vi "Estimate All Positions New.vi"(8 "Input AnchorArray":refnum<class "Anchor.lvclass">[](array[class]), 10 "Tag.lvclass":refnum<class "Tag.lvclass">) -> (2 "PositionCluster [tagID, x, y, anchorID, distances]":T2)   [LabVIEW 2014]
uses:
  Anchor/Anchor.lvclass
  Tag.lvclass
  Position.lvclass
panel:
  out "error out 3":errorcluster
  in  "error in (no error) 2":errorcluster
  out "error out 2":errorcluster
  out "TagID":dbl
  in  "error in (no error)":errorcluster
  out "Intersections":T1(array[cluster])
  # "This will be returned"
  # "Put intersection values in this control"
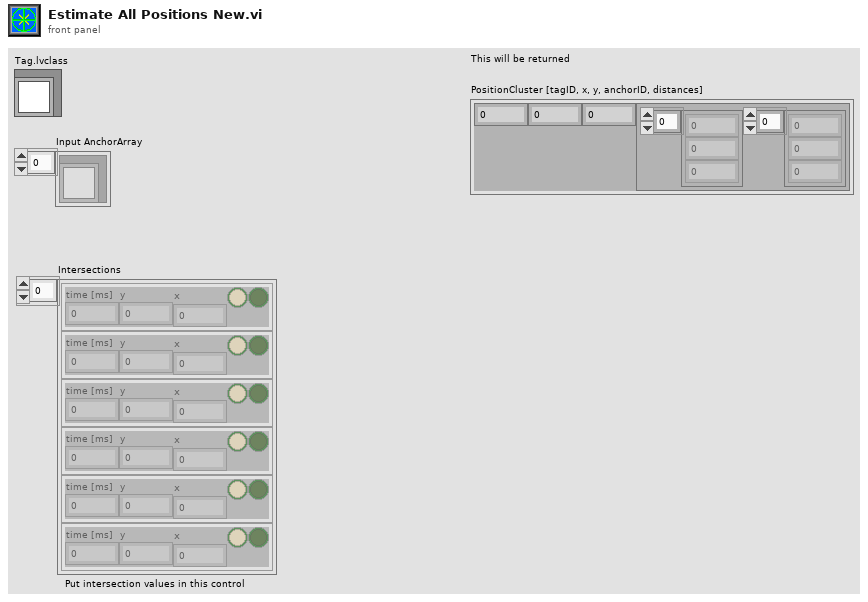
[diagram p1: front panel]
types:
  T1 = cluster{"time [ms]":dbl, "y":dbl, "x":dbl, "Fout":bool, "Goed":bool}[]
  T2 = cluster{"tagID":dbl, "X":dbl, "Y":dbl, "anchorIDDistanceCluster":cluster{"anchorIDArray":dbl[], "anchorDistanceArray":dbl[]}}
  T3 = cluster{"anchorIDArray":dbl[], "anchorDistanceArray":dbl[]}
  T4 = cluster{"Tag.lvclass":refnum<class "Tag.lvclass">, "Distance":dbl}[]
  T5 = cluster{"Time [ms]":dbl, "y":dbl, "x":dbl, "Fout":bool, "Goed":bool}[]
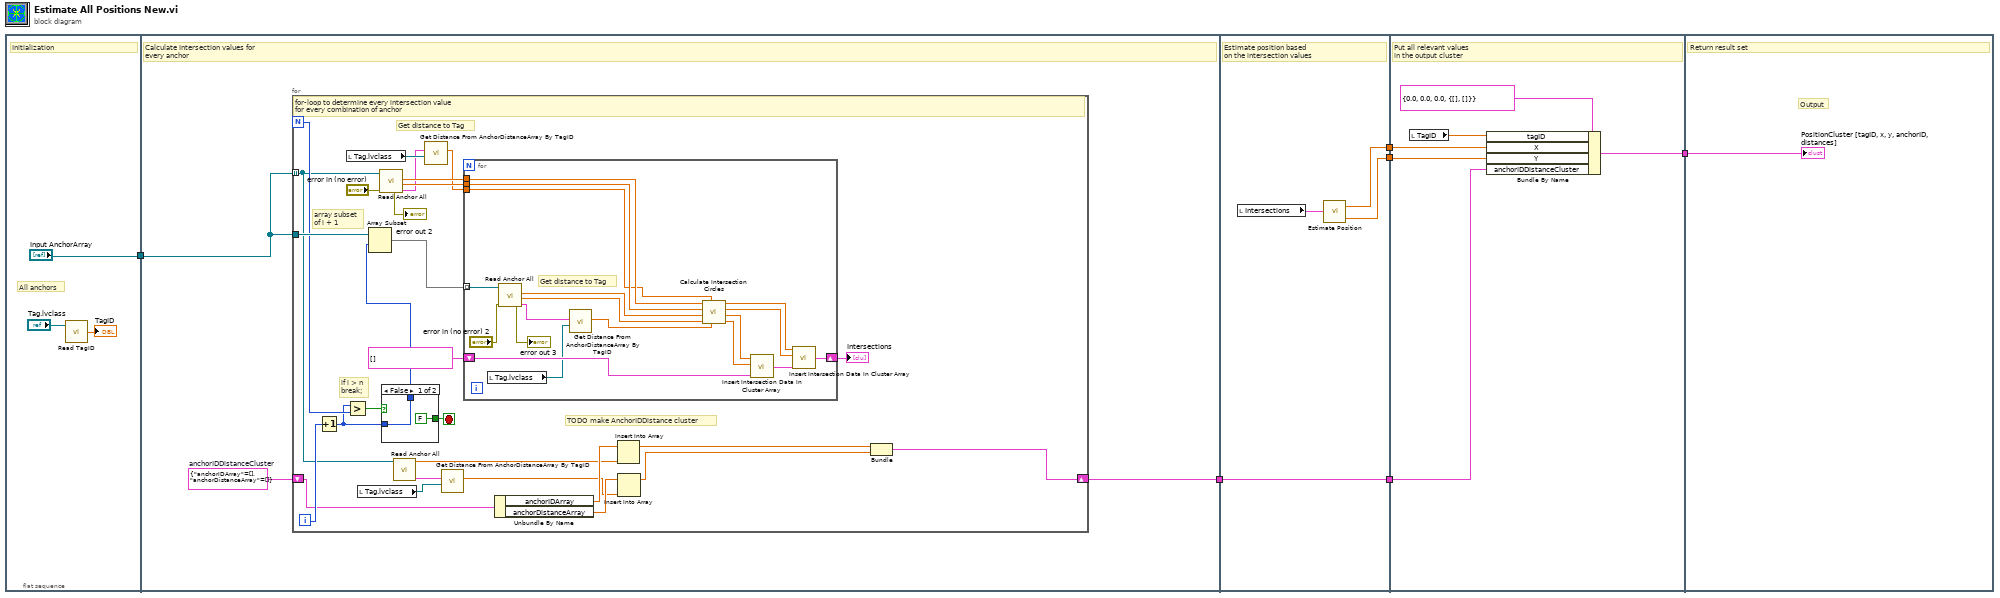
[diagram p0: block diagram]
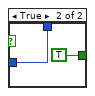
[diagram p2: hidden frame]
diagram:
  n1 = flat-sequence {
    tunnel: ["Input AnchorArray"] -> w6
    tunnel: w6 -> [w12]
    tunnel: [w10] -> w1
    tunnel: [w65] -> w5
    tunnel: [w64] -> w4
    tunnel: [w63] -> w2
    tunnel: w1 -> [w63]
    tunnel: w5 -> [w70]
    tunnel: w4 -> [w69]
    tunnel: [w68] -> w3
    tunnel: w2 -> [w67]
    tunnel: w3 -> [w73]
    frame #0 {
      # "All anchors"
      # "Initialization"
      n2 = call-dynamic "Read TagID.vi"("Tag in"="Tag.lvclass") -> ("TagID"=→"TagID":dbl)  [unwired: 1 in, 2 out]
    }
    frame #1 {
      w11 = T3 {"anchorIDArray"=[], "anchorDistanceArray"=[]}  # anchorIDDistanceCluster
      # "Calculate Intersection values for \nevery anchor"
      n3 = for {
        N -> [w28]
        tunnel: w12 -> [w36]
        tunnel: w12 -> [w23] mode=indexing
        shift-right: [w13] -> w10
        shift-left: w11 -> [w20]
        i -> [w32]
        stop <- w26 stop-if-true
        # "array subset\nof i + 1"
        # "TODO make AnchorIDDistance cluster"
        # "if i > n\nbreak;"
        # "Get distance to Tag"
        # "for-loop to determine every intersection value\nfor every combination of anchor"
        n4 = Increment(x=w32) -> (x+1=w25:i32)
        n5 = local read "Tag.lvclass"() -> (w31:refnum<class "Tag.lvclass">)
        n6 = Greater?(x=w25, y=w28) -> (0:w27:bool)
        n7 = local read "Tag.lvclass"() -> (w21:refnum<class "Tag.lvclass">)
        n8 = call "Read Anchor All.vi"("error in (no error)"="error in (no error)", "Anchor in"=w23) -> ("TagDistanceArray"=w30:T4, "AnchorY"=w33:dbl, "AnchorX"=w34:dbl, "error out"=→"error out 2":errorcluster)  [unwired: 4 in, 2 out]
        n9 = case shown="False" w27 {
          tunnel: [FALSE TRUE] -> w26
          tunnel: w25 -> [w41 w43]
          tunnel: [w41 w43] -> w24
          frame False {
          }
          frame True {
          }
        }
        n10 = Array Subset(array=w36, index=w24) -> (w35:refnum<class "Anchor.lvclass">[])  [unwired: 1 in]
        n11 = call "Read Anchor All.vi"("Anchor in"=w23) -> ("TagDistanceArray"=w22:T4, "AnchorID"=w17:dbl)  [unwired: 5 in, 4 out]
        n12 = call "Get Distance From AnchorDistanceArray By TagID.vi"("Tag.lvclass"=w31, "Input TagDistanceArray"=w30) -> ("Distance"=w29:dbl)  [unwired: 9 in]
        n13 = call "Get Distance From AnchorDistanceArray By TagID.vi"("Tag.lvclass"=w21, "Input TagDistanceArray"=w22) -> ("Distance"=w16:dbl)  [unwired: 9 in]
        n14 = for {
          shift-right: [w62] -> w40
          shift-left: T1 [] ("Intersections 2") -> [w61]
          tunnel: w35 -> [w59] mode=indexing
          tunnel: w34 -> [w58]
          tunnel: w33 -> [w57]
          tunnel: w29 -> [w45]
          # "Get distance to Tag"
          n15 = local read "Tag.lvclass"() -> (w47:refnum<class "Tag.lvclass">)
          n16 = call "Read Anchor All.vi"("error in (no error)"="error in (no error) 2", "Anchor in"=w59) -> ("TagDistanceArray"=w48:T4, "AnchorY"=w55:dbl, "AnchorX"=w56:dbl, "error out"=→"error out 3":errorcluster)  [unwired: 4 in, 2 out]
          n17 = call "Get Distance From AnchorDistanceArray By TagID.vi"("Tag.lvclass"=w47, "Input TagDistanceArray"=w48) -> ("Distance"=w46:dbl)  [unwired: 9 in]
          n18 = call "Calculate Intersection Circles.vi"("r2"=w46, "r1"=w45, "d"=w55, "c"=w56, "b"=w57, "a"=w58) -> ("y2"=w49:dbl, "x2"=w50:dbl, "y1"=w51:dbl, "x1"=w52:dbl)  [unwired: 2 in]
          n19 = call "Insert Intersection Data In Cluster Array.vi"("ClusterArray"=w61, "Y"=w49, "X"=w50) -> ("Intersections"=w60:T5)  [unwired: 1 in]
          n20 = call "Insert Intersection Data In Cluster Array.vi"("ClusterArray"=w60, "Y"=w51, "X"=w52) -> ("Intersections"=w62:T5)  [unwired: 1 in]
        }
        "Intersections" <- w40
        n21 = Unbundle By Name(w20) -> ("anchorIDArray"=w19:dbl[], "anchorDistanceArray"=w18:dbl[])
        n22 = Insert Into Array(array=w19, new element=w17) -> (w15:dbl[])  [unwired: 1 in]
        n23 = Insert Into Array(array=w18, new element=w16) -> (w14:dbl[])  [unwired: 1 in]
        n24 = Bundle("anchorIDArray"=w15, "anchorDistanceArray"=w14) -> (w13:T3)  [unwired: 1 in]
      }
    }
    frame #2 {
      # "Estimate position based\non the intersection values"
      n25 = local read "Intersections"() -> (w66:T1)
      n26 = call "Estimate Position.vi"("Intersections"=w66) -> ("X"=w65:dbl, "Y"=w64:dbl)
    }
    frame #3 {
      # "Put all relevant values\nin the output cluster"
      n27 = local read "TagID"() -> (w71:dbl)
      n28 = Bundle By Name(cluster=T2 {"tagID"=0.0, "X"=0.0, "Y"=0.0, "anchorIDDistanceCluster"={"anchorIDArray"=[], "anchorDistanceArray"=[]}} ("PositionCluster [tagID, x, y, anchorID, distances] 2"), "tagID"=w71, "X"=w70, "Y"=w69, "anchorIDDistanceCluster"=w67) -> (w68:T2)
    }
    frame #4 {
      # "Output"
      # "Return result set"
      "PositionCluster [tagID, x, y, anchorID, distances]" <- w73
    }
  }
